vi "Generate Report as INI Section.vi"(7 "Parameters":variant, 8 "error in (no error)":errorcluster, 9 "Results":variant, 10 "Refnum in":T1, 11 "Analyze Fluence in":refnum<class "Analyze Fluence.lvclass">) -> (0 "error out":errorcluster, 2 "Refnum out":T1, 3 "Analyze Fluence out":refnum<class "Analyze Fluence.lvclass">)   [LabVIEW 2020, in "Analyze.lvlib" / "Analyze Fluence.lvclass"]
uses:
  Analyze Fluence.lvclass
  <vilib>/Utility/config.llb/Config Data RefNum.ctl
  Fluence Info.ctl
  <vilib>/Utility/config.llb/Write Key (Double).vi
  <vilib>/Utility/config.llb/Write Key (I32).vi
  <vilib>/Utility/config.llb/NI_LVConfig.lvlib
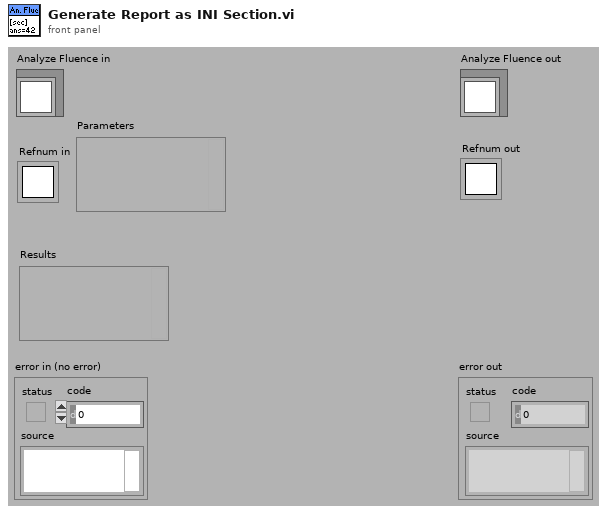
[diagram p1: front panel]
types:
  T1 = typedef "NI_LVConfig.lvlib/Config Data RefNum.ctl" = refnum<k1>
  T2 = typedef "Analyze.lvlib/Analyze Fluence.lvclass/Fluence Info.ctl" = cluster{"Fluence J/cm^2":dbl, "Energy in Area":dbl, "max value":i64, "Max fluence area":cluster{"Left":i32, "Top":i32, "Right":i32, "Bottom":i32}}
  T3 = cluster{"Left":i32, "Top":i32, "Right":i32, "Bottom":i32}
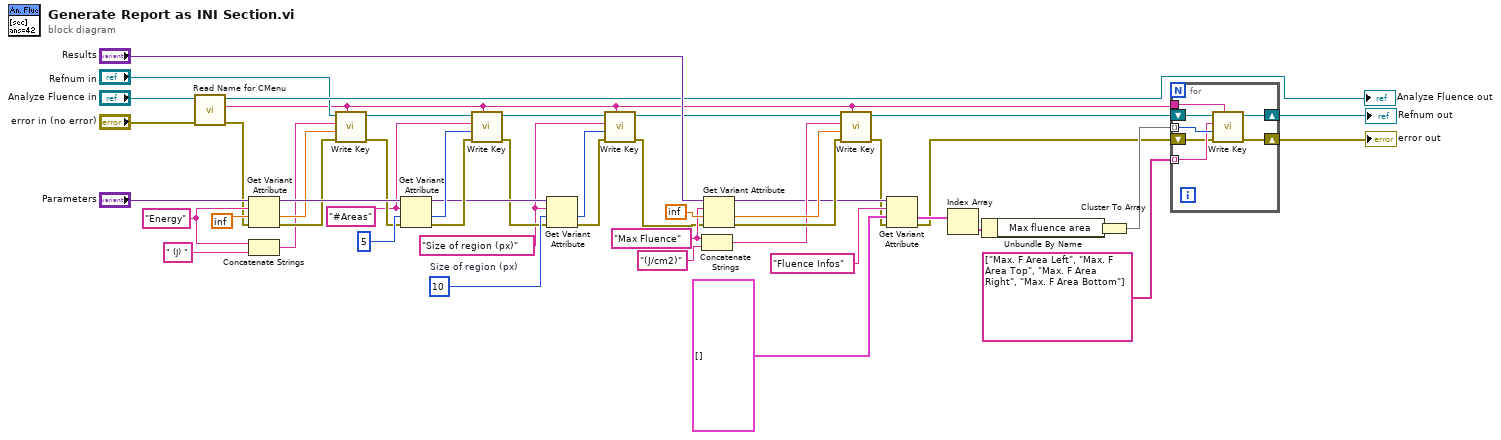
[diagram p0: block diagram]
diagram:
  w4 = "Size of region (px)" ("name")
  w7 = 10  # Size of region (px)
  w25 = "#Areas" ("name")
  w35 = "Energy" ("name")
  w45 = "Max Fluence" ("name")
  n1 = call-dynamic "Read Name for CMenu.vi"("error in (no error)"="error in (no error)", "Analyze BaseClass in"="Analyze Fluence in") -> ("error out"=w33:errorcluster, "Name for Context menu"=w9:string, "Analyze BaseClass out"=→"Analyze Fluence out":refnum<class "Analyze Fluence.lvclass">)  [unwired: 7 in]
  n2 = Get Variant Attribute(Variant="Parameters", name=w35, default value (empty Variant)=inf, error in=w33) -> (duplicate Variant=w40:variant, value=w36:dbl, error out=w32:errorcluster)  [unwired: 1 out]
  n3 = Concatenate Strings(w35, " (J) " ("string")) -> (w31:string)
  n4 = call-poly <vilib>:"Write Key.vi"("section"=w9, "error in (no error)"=w32, "value"=w36, "key"=w31, "refnum"="Refnum in") -> ("error out"=w28:errorcluster, "refnum out"=w29:T1)  [unwired: 4 in, 1 out]
  n5 = Get Variant Attribute(Variant=w40, name=w25, default value (empty Variant)=5, error in=w28) -> (duplicate Variant=w6:variant, value=w26:i32, error out=w27:errorcluster)  [unwired: 1 out]
  n6 = call-poly <vilib>:"Write Key.vi"("section"=w9, "error in (no error)"=w27, "value"=w26, "key"=w25, "refnum"=w29) -> ("error out"=w5:errorcluster, "refnum out"=w10:T1)  [unwired: 4 in, 1 out]
  n7 = Get Variant Attribute(Variant=w6, name=w4, default value (empty Variant)=w7, error in=w5) -> (value=w3:i32, error out=w2:errorcluster)  [unwired: 2 out]
  n8 = call-poly <vilib>:"Write Key.vi"("section"=w9, "error in (no error)"=w2, "value"=w3, "key"=w4, "refnum"=w10) -> ("error out"=w1:errorcluster, "refnum out"=w8:T1)  [unwired: 4 in, 1 out]
  n9 = Concatenate Strings(w45, "(J/cm2)" ("string")) -> (w24:string)
  n10 = Get Variant Attribute(Variant="Results", name=w45, default value (empty Variant)=inf, error in=w1) -> (duplicate Variant=w23:variant, value=w42:dbl, error out=w41:errorcluster)  [unwired: 1 out]
  n11 = call-poly <vilib>:"Write Key.vi"("section"=w9, "error in (no error)"=w41, "value"=w42, "key"=w24, "refnum"=w8) -> ("error out"=w14:errorcluster, "refnum out"=w16:T1)  [unwired: 4 in, 1 out]
  n12 = Get Variant Attribute(Variant=w23, name="Fluence Infos", default value (empty Variant)=T2[] [] ("fluence infos"), error in=w14) -> (value=w20:T2[], error out=w13:errorcluster)  [unwired: 2 out]
  n13 = Index Array(array=w20) -> (element=w19:T2)  [unwired: 1 in]
  n14 = Unbundle By Name(w19) -> ("Max fluence area"=w18:T3)
  n15 = Cluster To Array(cluster=w18) -> (array=w17:i32[])
  n16 = for {
    tunnel: w17 -> [w56] mode=indexing
    shift-right: [w54] -> w12
    shift-left: w16 -> [w55]
    tunnel: string[] ["Max. F Area Left", "Max. F Area Top", "Max. F Area Right", "Max. F Area Bottom"] -> [w53] mode=indexing
    shift-right: [w51] -> w11
    shift-left: w13 -> [w52]
    tunnel: w9 -> [w50]
    n17 = call-poly <vilib>:"Write Key.vi"("section"=w50, "error in (no error)"=w52, "value"=w56, "key"=w53, "refnum"=w55) -> ("error out"=w51:errorcluster, "refnum out"=w54:T1)  [unwired: 4 in, 1 out]
  }
  "error out" <- w11
  "Refnum out" <- w12
